vi "String to first letter lowercase 2(SubVI).vi"(6 "Couleur carré 2":string[](array[string]), 9 "Couleur carré 3":string[](array[string]), 10 "Couleur carré 1":string[](array[string]), 11 "Couleur carré 4":string[](array[string])) -> (1 "String 4":string, 2 "String 3":string, 3 "String 2":string, 4 "String":string)   [LabVIEW 2019]
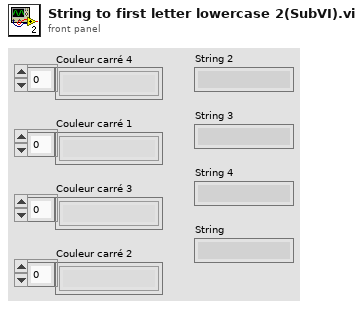
[diagram p1: front panel]
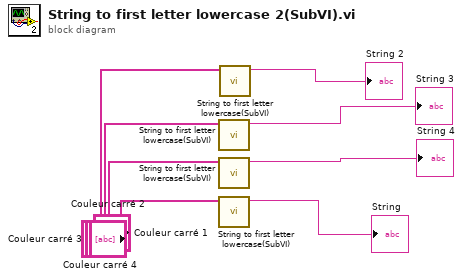
[diagram p0: block diagram]
diagram:
  n1 = call "String to first letter lowercase(SubVI).vi"("Couleur carré"="Couleur carré 3") -> ("String"=→"String 3":string)  [unwired: 10 in]
  n2 = call "String to first letter lowercase(SubVI).vi"("Couleur carré"="Couleur carré 2") -> ("String"=→"String 4":string)  [unwired: 10 in]
  n3 = call "String to first letter lowercase(SubVI).vi"("Couleur carré"="Couleur carré 1") -> ("String"=→"String":string)  [unwired: 10 in]
  n4 = call "String to first letter lowercase(SubVI).vi"("Couleur carré"="Couleur carré 4") -> ("String"=→"String 2":string)  [unwired: 10 in]
